vi "Render.vi"(8 "error in (no error)":errorcluster, 10 "String in":string, 11 "Bold in":refnum<class "Italic.lvclass">) -> (0 "error out":errorcluster, 2 "String out":string, 3 "Bold out":refnum<class "Italic.lvclass">)   [LabVIEW 2021, in "Markdown.lvlib" / "Italic.lvclass"]
uses:
  Italic.lvclass
  C:/GitHub/Markdown/src/Markdown/Markdown.lvclass
  ItalicTag.vi
  Italic.lvclass/Italic.ctl
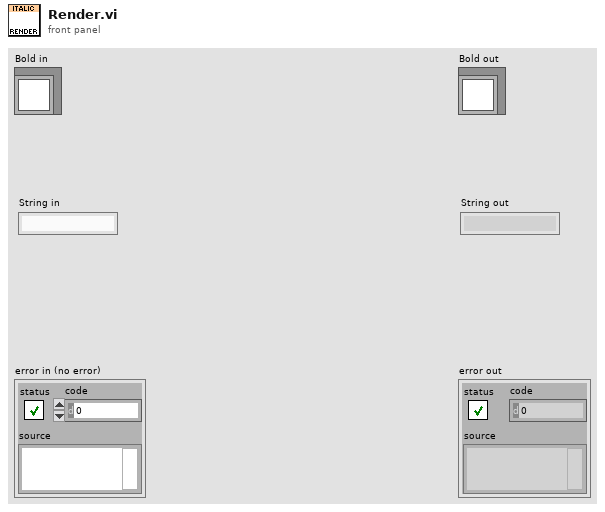
[diagram p1: front panel]
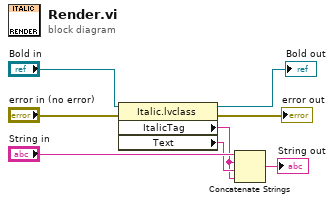
[diagram p0: block diagram]
diagram:
  n1 = property class="Italic.lvclass"(reference="Bold in", error in="error in (no error)") -> (reference out=→"Bold out":refnum<class "Italic.lvclass">, error out=→"error out":errorcluster, "ItalicTag"=w6:string, "Text"=w7:string)
  n2 = Concatenate Strings("String in", w6, w7, w6) -> (→"String out":string)
